vi "CallSubMenu.vi"(0 "Menu in":refnum<class "Menu.lvclass">, 1 "User Event":refnum<user-event>, 3 "CtrlRef":refnum<vi>, 5 "Selected Area":T2, 9 "Selected Tag":string, 11 "error in (no error)":errorcluster, 12 "SubMenu":bool, 13 "ContextMenu":bool, 14 "Coords":T1) -> (4 "Menu out":refnum<class "Menu.lvclass">, 15 "error out":errorcluster)   [LabVIEW 2021, in "Menu.lvlib" / "Menu.lvclass"]
uses:
  Menu.lvclass
  <vilib>/Utility/miscctls.llb/LVPoint32TypeDef.ctl
  SubMenu.vi
  <vilib>/Utility/error.llb/Error Cluster From Error Code.vi
  <vilib>/ErrorRing/Error Ring.xnode
  Menu.lvclass/Menu.ctl
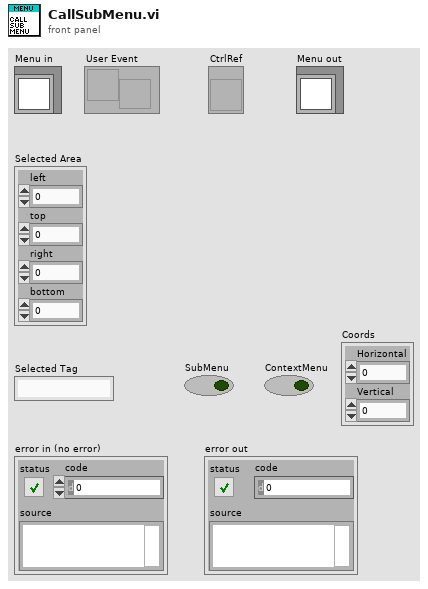
[diagram p1: front panel]
types:
  T1 = typedef "LVPoint32TypeDef.ctl" = cluster{"Horizontal":i32, "Vertical":i32}
  T2 = cluster{"left":i16, "top":i16, "right":i16, "bottom":i16}
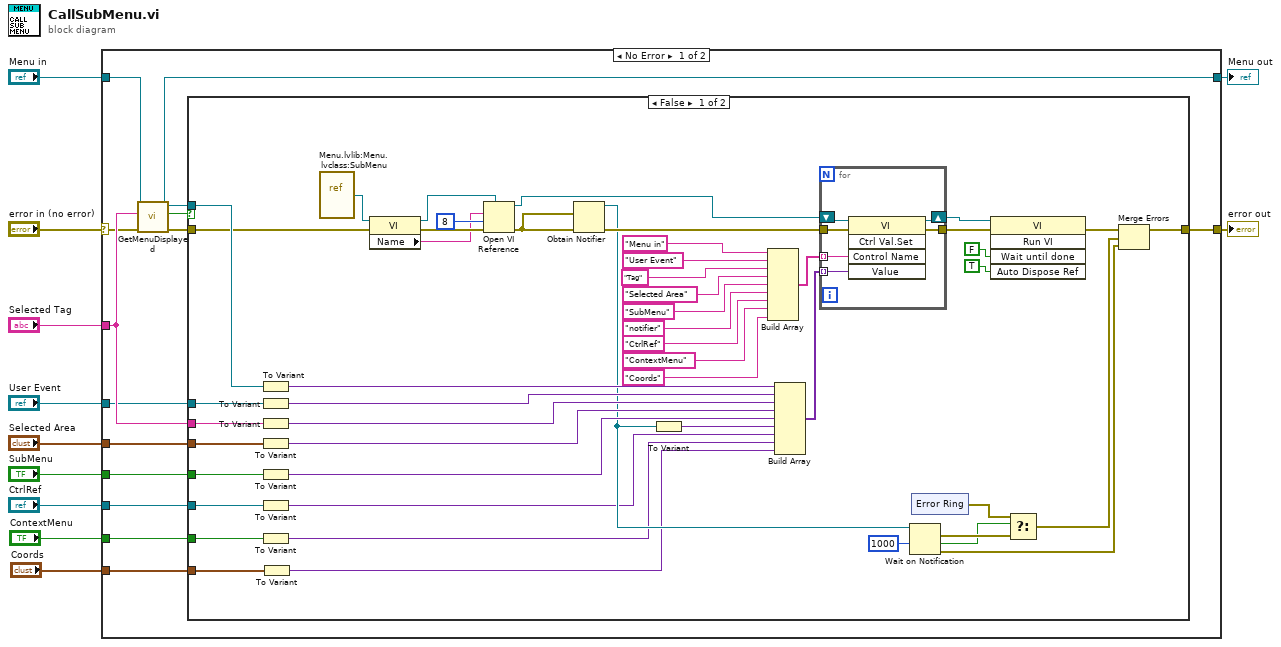
[diagram p0: block diagram]
diagram:
  n1 = case shown="No Error" "error in (no error)" {
    selector: "error in (no error)" -> [w18 w86]
    tunnel: [w24 w86] -> w11
    tunnel: "Selected Area" -> [w23 _]
    tunnel: "SubMenu" -> [w22 _]
    tunnel: "Menu in" -> [w21 w87]
    tunnel: [w20 w87] -> w7
    tunnel: "Selected Tag" -> [w19 _]
    tunnel: "User Event" -> [w16 _]
    tunnel: "CtrlRef" -> [w14 _]
    tunnel: "ContextMenu" -> [w13 _]
    tunnel: "Coords" -> [w12 _]
    frame No Error {
      n2 = call "GetMenuDisplayed.vi"("error in (no error)"=w18, "Tag"=w19, "Menu in"=w21) -> ("error out"=w17:errorcluster, "Displayed?"=w15:bool, "Menu out"=w20:refnum<class "Menu.lvclass">)  [unwired: 6 in]
      n3 = case shown="False" w15 {
        tunnel: [w68 w85] -> w24
        tunnel: w23 -> [w74 _]
        tunnel: w22 -> [w73 _]
        tunnel: w20 -> [w72 _]
        tunnel: w19 -> [w71 _]
        tunnel: w17 -> [w70 w85]
        tunnel: w16 -> [w69 _]
        tunnel: w14 -> [w32 _]
        tunnel: w13 -> [w30 _]
        tunnel: w12 -> [w26 _]
        frame False {
          n4 = To Variant(anything=w72) -> (Variant=w53:variant)
          n5 = To Variant(anything=w69) -> (Variant=w51:variant)
          n6 = To Variant(anything=w71) -> (Variant=w52:variant)
          n7 = To Variant(anything=w74) -> (Variant=w50:variant)
          n8 = To Variant(anything=w73) -> (Variant=w49:variant)
          n9 = To Variant(anything=w32) -> (Variant=w31:variant)
          n10 = To Variant(anything=w30) -> (Variant=w29:variant)
          n11 = To Variant(anything=w26) -> (Variant=w25:variant)
          n12 = vi-ref "Menu.lvlib:Menu.lvclass:SubMenu.vi"() -> (w63:refnum<vi>)
          n13 = property class="VI"(reference=w63, error in=w70) -> (reference out=w66:refnum<vi>, error out=w67:errorcluster, "Name"=w64:string)
          n14 = Open VI Reference(type specifier VI Refnum (for type only)=w66, vi path=w64, options=8, error in (no error)=w67) -> (vi reference=w46:refnum<vi>, error out=w42:errorcluster)  [unwired: 2 in]
          n15 = Obtain Notifier(notification data type=w42, error in (no error)=w42) -> (notifier out=w41:refnum<notifier>, error out=w43:errorcluster)  [unwired: 2 in, 1 out]
          n16 = To Variant(anything=w41) -> (Variant=w44:variant)
          n17 = Build Array("Menu in" ("Control Name"), "User Event" ("Control Name"), "Tag" ("Control Name"), "Selected Area" ("Control Name"), "SubMenu" ("Control Name"), "notifier" ("Control Name"), "CtrlRef", "ContextMenu", "Coords") -> (w47:string[])
          n18 = Build Array(w53, w51, w52, w50, w49, w44, w31, w29, w25) -> (w48:variant[])
          n19 = for {
            tunnel: [w83] -> w59
            tunnel: w48 -> [w82] mode=indexing
            tunnel: w47 -> [w81] mode=indexing
            tunnel: w43 -> [w79]
            shift-right: [w84] -> w60
            shift-left: w46 -> [w80]
            n20 = invoke class="VI" method="Ctrl Val.Set"(reference=w80, error in=w79, "Control Name"=w81, "Value"=w82) -> (reference out=w84:refnum<vi>, error out=w83:errorcluster)  [unwired: 1 in, 3 out]
          }
          n21 = Wait on Notification(notifier=w41, timeout in ms (-1)=1000) -> (notification=w36:errorcluster, timed out?=w35:bool, error out=w39:errorcluster)  [unwired: 2 in, 1 out]
          n22 = xnode "Error Ring"() -> ("error out"=w34:errorcluster)
          n23 = invoke class="VI" method="Run VI"(reference=w60, error in=w59, "Wait until done"=FALSE ("Wait Until Done"), "Auto Dispose Ref"=TRUE ("Auto Dispose Reference")) -> (error out=w38:errorcluster)  [unwired: 1 in, 4 out]
          n24 = Select(t=w34, s=w35, f=w36) -> (s? t:f=w37:errorcluster)
          n25 = Merge Errors(w38, w37, w39) -> (w68:errorcluster)
        }
        frame True {
        }
      }
    }
    frame Error {
    }
  }
  "Menu out" <- w7
  "error out" <- w11
